vi "Write Device Channel Names.vi"(8 "error in (no error)":errorcluster, 10 "Device Channel Names":string[](array[string]), 11 "2525 in":refnum<class "2525.lvclass">) -> (0 "error out":errorcluster, 3 "2525 out":refnum<class "2525.lvclass">)   [LabVIEW 2019, in "2525.lvlib" / "2525.lvclass"]
uses:
  Library/2525.lvclass
  Library/2525.lvclass/2525.ctl
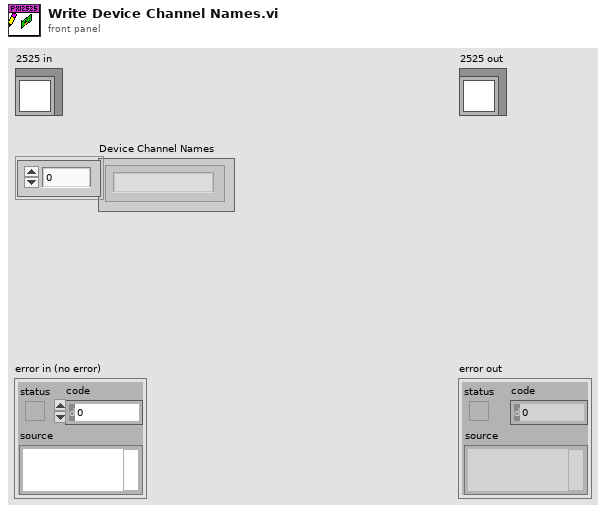
[diagram p1: front panel]
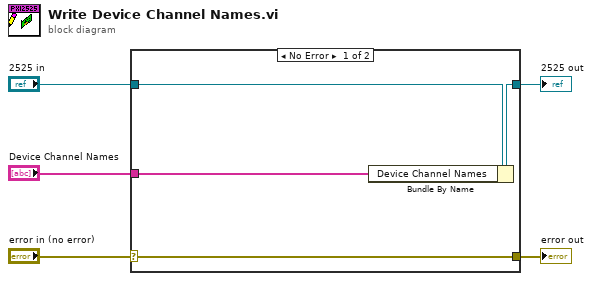
[diagram p0: block diagram]
diagram:
  n1 = case shown="No Error" "error in (no error)" {
    selector: "error in (no error)" -> [w9 w10]
    tunnel: [w9 w10] -> w4
    tunnel: [w7 w11] -> w2
    tunnel: "2525 in" -> [w8 w11]
    tunnel: "Device Channel Names" -> [w6 _]
    frame No Error {
      n2 = Bundle By Name(cluster=w8, "Device Channel Names"=w6) -> (w7:refnum<class "2525.lvclass">)
    }
    frame Error {
    }
  }
  "error out" <- w4
  "2525 out" <- w2
